vi "Dialog - Edit Size.vi"(0 "Height":u32, 1 "Queue":refnum<queue>, 5 "Width":u32, 7 "CtrlRef":refnum<vi>) -> ()   [LabVIEW 2011]
panel:
  in  "Apply to All":bool
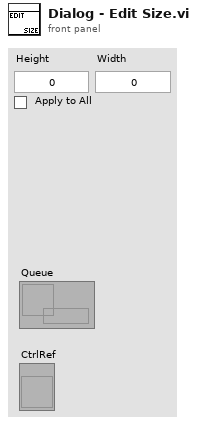
[diagram p1: front panel]
types:
  T1 = cluster{"CtrlRef":refnum<vi>, cluster{"Width":u32, "Height":u32}}
  T2 = enum8{"Enabled", "Disabled", "Disabled and Grayed Out"}
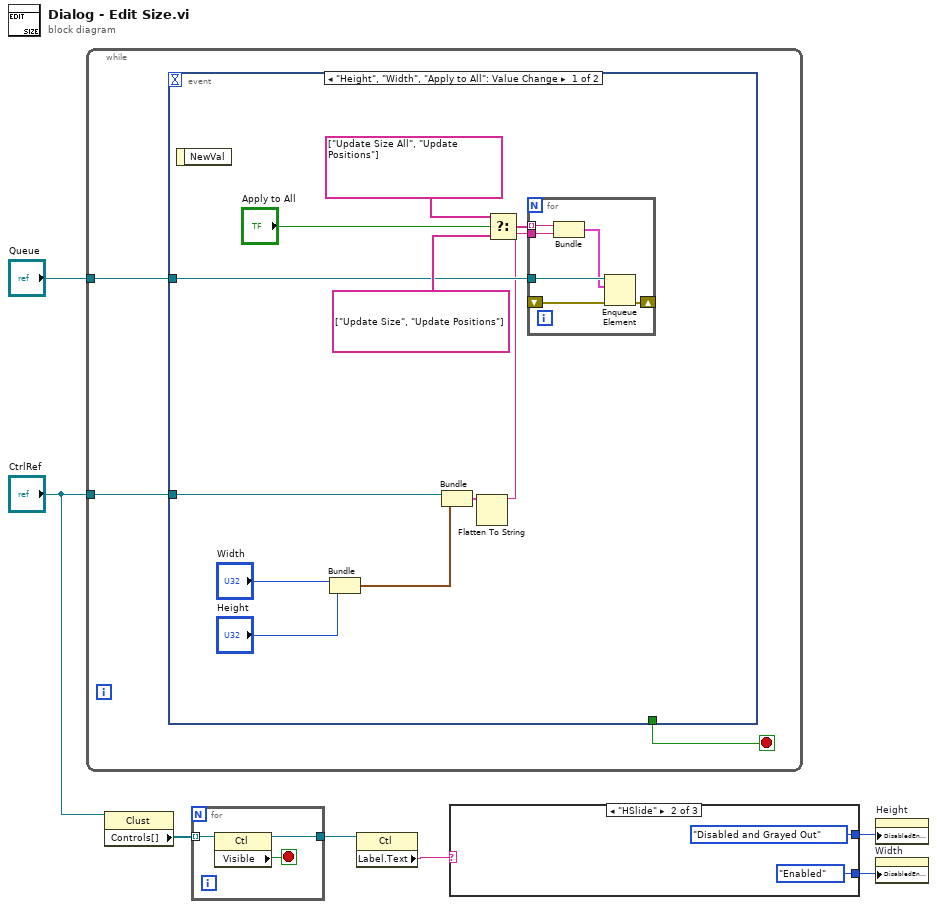
[diagram p0: block diagram]
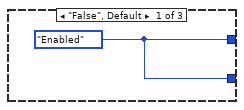
[diagram p2: hidden frame]
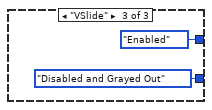
[diagram p3: hidden frame]
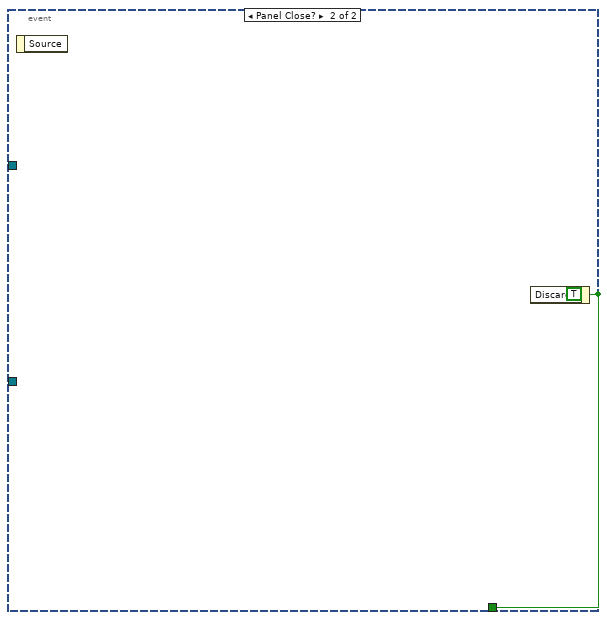
[diagram p4: hidden frame]
diagram:
  n1 = while {
    tunnel: "Queue" -> [w9]
    tunnel: "CtrlRef" -> [w8]
    stop <- w10 stop-if-true
    n2 = event shown="[0] \"Height\", \"Width\", \"Apply to All\": Value Change" {
      selector: _ -> [_ _]
      dyn-events: _ -> [_ _]
      timeout: _ -> [_ _]
      tunnel: [_ w28] -> w10
      tunnel: w9 -> [w13 _]
      tunnel: w8 -> [w21 _]
      event "Height", "Width", "Apply to All": Value Change {
        n3 = event-data() -> ()  [unwired: 1 in, 1 out]
        n4 = Bundle("Width"="Width", "Height"="Height") -> (w18:cluster{"Width":u32, "Height":u32})  [unwired: 1 in]
        n5 = Bundle("CtrlRef"=w21, w18) -> (w17:T1)  [unwired: 1 in]
        n6 = Flatten To String(anything=w17) -> (data string=w11:string)  [unwired: 3 in, 2 out]
        n7 = Select(t=string[] ["Update Size All", "Update Positions"], s="Apply to All", f=string[] ["Update Size", "Update Positions"]) -> (s? t:f=w12:string[])
        n8 = for {
          tunnel: w12 -> [w25] mode=indexing
          shift-right: [w26] -> _
          shift-left: _ -> [w27]
          tunnel: w13 -> [w24]
          tunnel: w11 -> [w22]
          n9 = Bundle(w25, "data string"=w22) -> (w23:cluster{string, "data string":string})  [unwired: 1 in]
          n10 = Enqueue Element(queue=w24, element=w23, error in (no error)=w27) -> (error out=w26:errorcluster)  [unwired: 1 in, 2 out]
        }
      }
      event Panel Close? {
        w28 = TRUE ("Discard?")
        n11 = event-data() -> ()  [unwired: 1 in, 1 out]
        n12 = event-data("Discard?"=w28) -> ()  [unwired: 1 in, 1 out]
      }
    }
  }
  n13 = property class="Clust"(reference="CtrlRef") -> ("Controls[]"=w7:refnum<vi>[])  [unwired: 1 in, 2 out]
  n14 = for {
    tunnel: w7 -> [w31] mode=indexing
    tunnel: [w29] -> w5
    stop <- w30 stop-if-true
    n15 = property class="Ctl"(reference=w31) -> (reference out=w29:refnum<vi>, "Visible"=w30:bool)  [unwired: 1 in, 1 out]
  }
  n16 = property class="Ctl"(reference=w5) -> ("Label.Text"=w4:string)  [unwired: 1 in, 2 out]
  n17 = case shown="\"HSlide\"" w4 {
    tunnel: [w32 T2."Disabled and Grayed Out" ("Disabled") T2."Enabled" ("Disabled")] -> w3
    tunnel: [w32 T2."Enabled" ("Disabled") T2."Disabled and Grayed Out" ("Disabled")] -> w2
    frame "False", Default {
      w32 = T2."Enabled" ("Disabled")
    }
    frame "HSlide" {
    }
    frame "VSlide" {
    }
  }
  n18 = property on="Height" class="DigNum (strict)"("DisabledEnum"=w3) -> ()  [unwired: 2 in, 2 out]
  n19 = property on="Width" class="DigNum (strict)"("DisabledEnum"=w2) -> ()  [unwired: 2 in, 2 out]
